vi "Lab Panel V6.00.vi"() -> ()   [LabVIEW 2017] (continued)
                      frame True {
                        n3712 = One Button Dialog(message="USB ERROR, program will be stopped.\nClose program, close windows, switch panel off\nand re power panel. If error persists seek help.") -> ()  [unwired: 1 in, 1 out]
                      }
                    }
                  }
                  frame True {
                  }
                }
              }
              frame #2 {
                # "end labview session"
                n3713 = case shown="True" w6464 {
                  tunnel: [_ TRUE] -> w6463
                  frame False {
                  }
                  frame True {
                    n3714 = call "sub vi - AI USB4704 (3)  Close Task v2.vi"() -> ()  [unwired: 16 in]
                  }
                }
                n3715 = Or(x=w6466, y="stop all") -> (x .or. y?=w6465:bool)
                n3716 = case shown="True" w6465 {
                  tunnel: w6463 -> [_ _]
                  frame False {
                  }
                  frame True {
                    n3717 = stacked-sequence {
                      frame #0 {
                        n3718 = global write "Global display 1.vi" "stop disp"(TRUE) -> ()
                      }
                      frame #1 {
                        n3719 = call "sub vi - AI USB4704 (3)  Close Task v2.vi"() -> ()  [unwired: 16 in]
                      }
                      frame #2 {
                        n3720 = Quit LabVIEW(quit? (T)=TRUE) -> ()
                      }
                    }
                  }
                }
              }
            }
          }
          frame #25 {
            n3721 = disable-structure shown="Enabled" {
              frame Disabled {
                n3722 = call <userlib>:"Periodic Trigger__ogtk.vi"("time (ms)"=u32 1500) -> ("Triggered"=w6479:bool)  [unwired: 12 in, 2 out]
                n3723 = case shown="True" w6479 {
                  frame False {
                  }
                  frame True {
                    n3724 = local read "Application Directory"() -> (w6481:path)
                    n3725 = control-ref of="This VI"() -> (w6490:refnum<vi>)
                    n3726 = control-ref of="Main Control"() -> (w6488:refnum<vi>)
                    n3727 = Bundle By Name(cluster=T24 {"Tab Ref"=refnum, "Values"=[]} ("Image Data"), "Tab Ref"=w6488, "Values"=i32[] [0, 2]) -> (w6486:T24)
                    n3728 = call "SaveWWWImages2.vi"("Image Data 2"=w6486, "Destination"=w6481, "VI in"=w6490) -> ()  [unwired: 9 in]
                    n3729 = control-ref of="LAB01 deg C"() -> (w6483:refnum<vi>)
                    n3730 = control-ref of="LAB01 AMPS"() -> (w6485:refnum<vi>)
                    n3731 = control-ref of="LAB01 VOLTS"() -> (w6484:refnum<vi>)
                    n3732 = Build Array(w6485, w6484, w6483) -> (w6482:refnum<vi>[])
                    n3733 = call "SaveWWWChartImages.vi"("Chart Refs"=w6482, "Destination"=w6481) -> ()  [unwired: 10 in]
                  }
                }
              }
              frame Enabled {
              }
            }
            n3734 = disable-structure shown="Enabled" {
              frame Disabled {
                n3735 = call <userlib>:"Periodic Trigger__ogtk.vi"("time (ms)"=u32 3000) -> ("Triggered"=w6471:bool)  [unwired: 12 in, 2 out]
                n3736 = case shown="True" w6471 {
                  frame False {
                  }
                  frame True {
                    n3737 = local read "Application Directory"() -> (w6474:path)
                    n3738 = control-ref of="This VI"() -> (w6475:refnum<vi>)
                    n3739 = control-ref of="Main Control"() -> (w6473:refnum<vi>)
                    n3740 = Bundle By Name(cluster=T24 {"Tab Ref"=refnum, "Values"=[]} ("Image Data"), "Tab Ref"=w6473, "Values"=i32[] [1, 5]) -> (w6476:T24)
                    n3741 = call "SaveWWWImages2.vi"("Image Data 2"=w6476, "Destination"=w6474, "VI in"=w6475) -> ()  [unwired: 9 in]
                  }
                }
              }
              frame Enabled {
              }
            }
          }
          frame #26 {
            n3742 = Tick Count (ms)() -> (millisecond timer value=w6493:u32)
            n3743 = Subtract(x=w6493, y=w6492) -> (x-y=→"Loop Time":u32)
          }
        }
        n3744 = node-c288() -> ()  [unwired: 1 in, 1 out]
        "loops" <- w379
      }
      n3745 = node-c288(w350) -> ()  [unwired: 1 out]
    }
  }
